vi "WSVCAP SHL FPGA LL Procedure I2C - Receive Byte.vi"(0 "Procedure Step":T1, 1 "Wait Ticks Remaining":u32, 5 "I2C Wait Ticks":u32, 7 "Read Bits Remaining":u8, 9 "Read Bytes Remaining":u8, 11 "error in (no error)":errorcluster, 13 "Socket Mask":u64 format="%012x", 14 "UUT Set (0/1)":u8) -> (3 "Wait Ticks Remaining Out":u32, 4 "Procedure Step Out":T1, 6 "Finished":bool, 8 "Read Bits Remaining Out":u8, 10 "Read Bytes Remaining Out":u8, 15 "error out":errorcluster)   [LabVIEW 2017]
uses:
  Type Defs/WSVCAP SHL Procedure Step Enum.ctl
  Type Defs/WSVCAP SHL FIFO Operation Enum.ctl
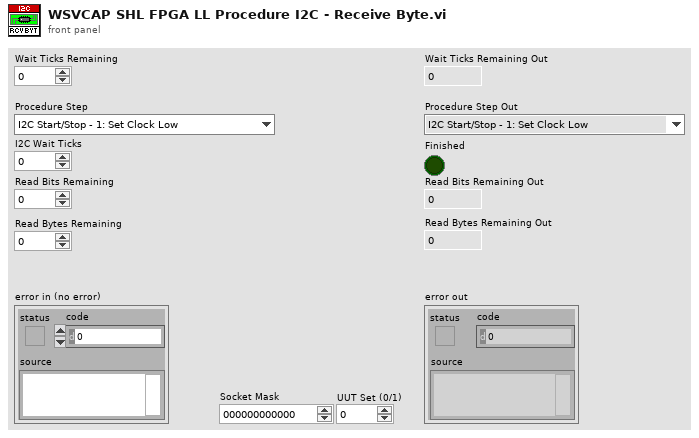
[diagram p1: front panel]
types:
  T1 = typedef "WSVCAP SHL Procedure Step Enum.ctl" = enum16{"I2C Start/Stop - 1: Set Clock Low", "I2C Start/Stop - 2: Wait", "I2C Start/Stop - 3: Set Data I", "I2C Start/Stop - 4: Wait", "I2C Start/Stop - 5: Set Clock High", "I2C Start/Stop - 6: Wait", "I2C Start/Stop - 7: Set Data II", "I2C Start/Stop - 8: Wait", "I2C Start/Stop - 9: Set Clock Low", "I2C Start/Stop - 10: Wait", "I2C Read ACK - 1: Set Clock High", "I2C Read ACK - 2: Wait", "I2C Read ACK - 3: Read ACK Bit", "I2C Read ACK - 4: Wait", "I2C Read ACK - 5: Set Clock Low", "I2C Read ACK - 6: Wait", "I2C Write ACK - 1: Write ACK Bit", "I2C Write ACK - 2: Wait", "I2C Write ACK - 3: Set Clock High", "I2C Write ACK - 4: Wait", "I2C Write ACK - 5: Set Clock Low", "I2C Write ACK - 6: Wait", "I2C Write ACK - 7: Set Data Low", "I2C Send Add - 1: Reset Bits Remaining", "I2C Send Add - 2: Set Data Bit", "I2C Send Add - 3: Wait", "I2C Send Add - 4: Set Clock High", "I2C Send Add - 5: Wait", "I2C Send Add - 6: Set Clock Low", "I2C Send Add - 7: Wait", "I2C Send Add - 8: Check Bits Remaining", "I2C Send Data - 1: Reset Bits Remaining", "I2C Send Data - 2: Load Write Bit from FIFO", "I2C Send Data - 3: Set Data Bit", "I2C Send Data - 4: Wait", "I2C Send Data - 5: Set Clock High", "I2C Send Data - 6: Wait", "I2C Send Data - 7: Set Clock Low", "I2C Send Data - 8: Wait", "I2C Send Data - 9: Check Bits Remaining", "I2C Receive Data - 1: Reset Bits Remaining", "I2C Receive Data - 2: Wait", "I2C Receive Data - 3: Set Clock High", "I2C Receive Data - 4: Wait", "I2C Receive Data - 5: Read Data Bit", "I2C Receive Data - 6: Wait", "I2C Receive Data - 7: Set Clock Low", "I2C Receive Data - 8: Wait", "I2C Receive Data - 9: Check Bits Remaining", "RFFE Send SSC - 1:Set Low", "RFFE Send SSC - 2:Wait", "RFFE Send SSC - 3:Set SDA High", "RFFE Send SSC - 4:Wait", "RFFE Send SSC - 5:Set SDA Low", "RFFE Send SSC - 6:Wait", "RFFE Send Data - 1:Set SCL High", "RFFE Send Data - 2:Wait", "RFFE Send Data - 3:Set SCL Low", "RFFE Send Data - 4:Wait", "RFFE Send Data - 5:Set SCL High (P)", "RFFE Send Data - 6:Wait", "RFFE Send Data - 7:Set SCL Low (P)", "RFFE Send Data - 8:Wait", "RFFE Send Data - 9:Set SCL High (BP)", "RFFE Send Data - 10:Wait", "RFFE Send Data - 11:Set SCL Low (BP)", "RFFE Send Data - 12:Wait", "RFFE Receive Data - 1:Set SCL High", "RFFE Receive Data - 2:Wait", "RFFE Receive Data - 3:Set SCL Low", "RFFE Receive Data - 4:Wait", "RFFE Receive Data - 5:Set SCL High (BP)", "RFFE Receive Data - 6:Wait", "RFFE Receive Data - 7:Set SCL Low (BP)", "RFFE Receive Data - 8:Wait", "RFFE Wait CMD Delay - 1:Wait", "RFFE Clear Lines - 1:Clear", "SRL Write Data - 1:Set SYNC High", "SRL Write Data - 2:Wait SYNC Delay", "SRL Write Data - 3:Set SYNC Low", "SRL Write Data - 4:Set SCLK High", "SRL Write Data - 5:Wait", "SRL Write Data - 6:Set SCLK Low", "SRL Write Data - 7:Wait", "SRL Write Data - 8:Set SYNC High", "SRL Wait CMD Delay - 1:Wait", "SRL Clear Lines - 1:Clear"}
  T2 = typedef "WSVCAP SHL FIFO Operation Enum.ctl" = enum16{"Create FIFO/Memory", "Get Write FIFO Status", "Get Read FIFO Status", "Put Element in Write", "Put Element in Read", "Get Element from Write", "Get Element from Read"}
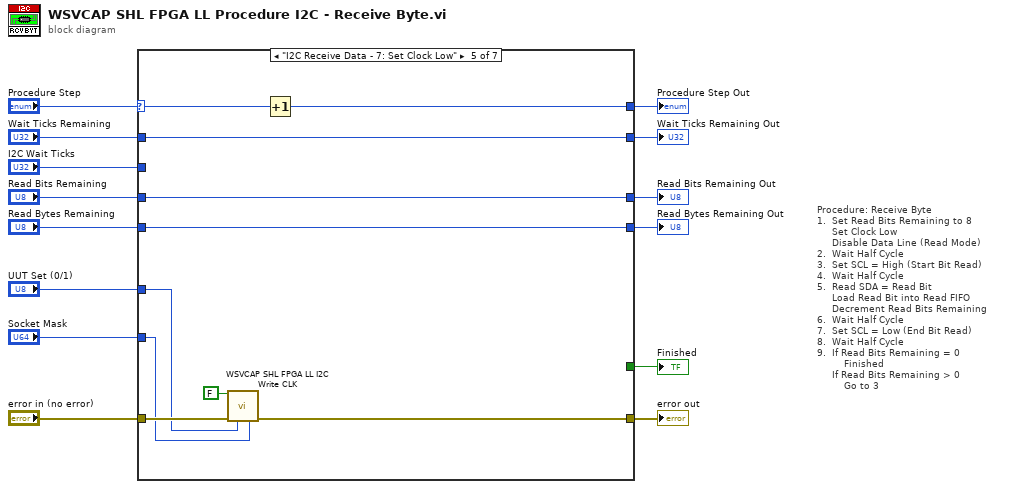
[diagram p0: block diagram]
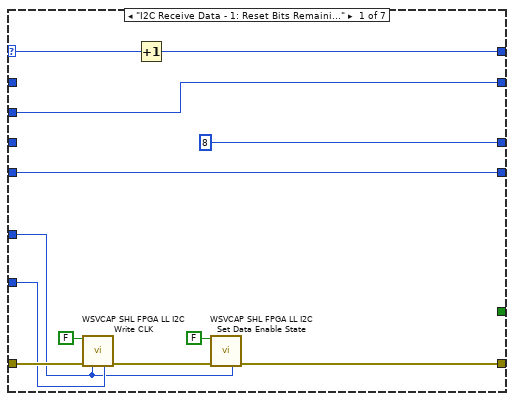
[diagram p2: hidden frame]
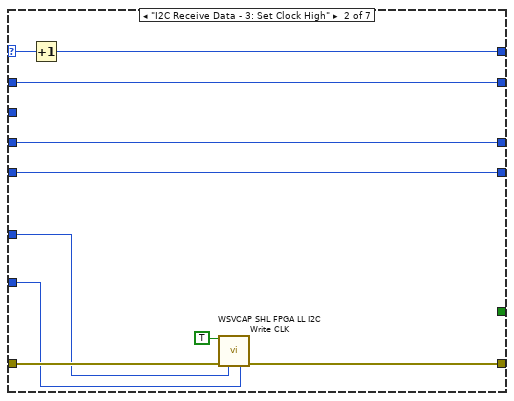
[diagram p3: hidden frame]
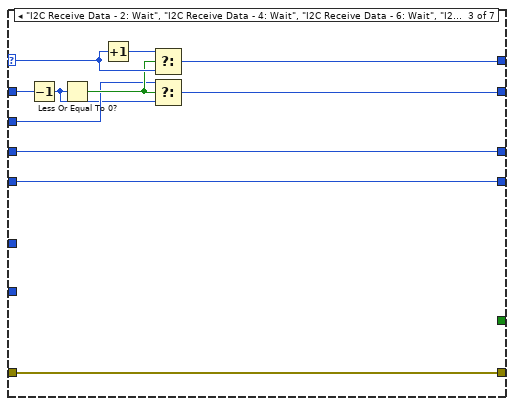
[diagram p4: hidden frame]
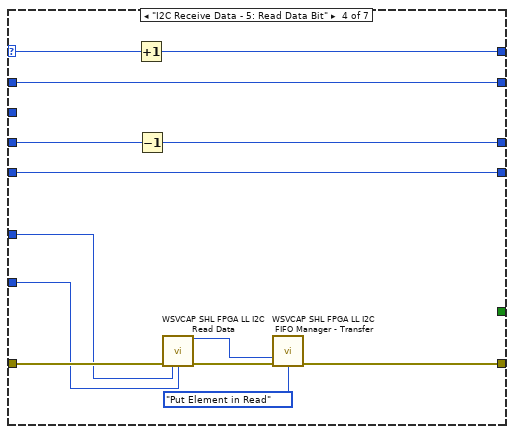
[diagram p5: hidden frame]
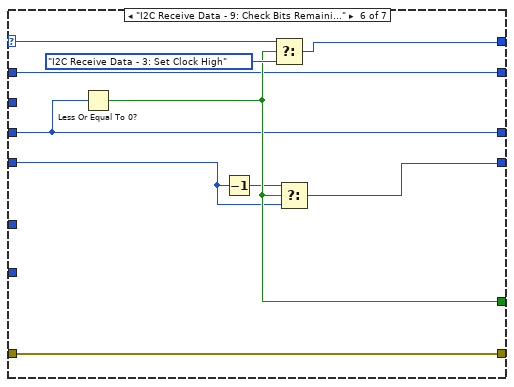
[diagram p6: hidden frame]
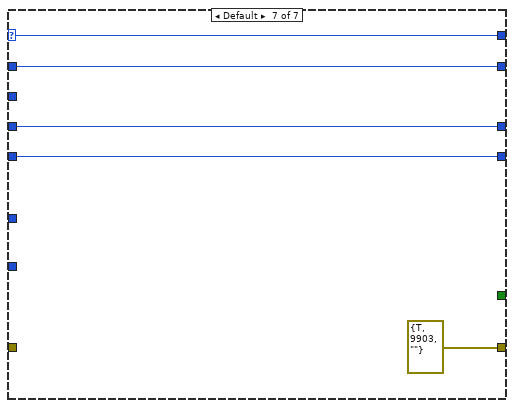
[diagram p7: hidden frame]
diagram:
  # "Procedure: Receive Byte\n1.  Set Read Bits Remaining to 8 \n     Set Clock Low\n     Disable Data Line (Read Mode)\n2.  Wait Half Cycle\n3.  Set SCL = High (Start Bit Read)\n4.  Wait Half Cycle\n5.  Read SDA = Read Bit\n     Load Read Bit into Read FIFO\n     Decrement Read Bits Remaining\n6.  Wait Half Cycle\n7.  Set SCL = Low (End Bit Read)\n8.  Wait Half Cycle\n9.  If Read Bits Remaining = 0\n         Finished\n     If Read Bits Remaining > 0\n         Go to 3"
  n1 = case shown="\"I2C Receive Data - 7: Set Clock Low\"" "Procedure Step" {
    selector: "Procedure Step" -> [w24 w34 w46 w59 w67 w75 w84]
    tunnel: [w22 w35 w44 w57 w69 w80 errorcluster {"status"=TRUE, "code"=9903, "source"=""} ("error IO")] -> w13
    tunnel: "error in (no error)" -> [w26 w36 w44 w60 w70 w80 _]
    tunnel: "Wait Ticks Remaining" -> [_ w30 w47 w50 w64 w72 w83]
    tunnel: "I2C Wait Ticks" -> [w17 _ w42 _ _ _ _]
    tunnel: "Read Bits Remaining" -> [_ w29 w38 w54 w63 w71 w82]
    tunnel: [_ _ _ _ _ w78 _] -> w12
    tunnel: "Socket Mask" -> [w20 w32 _ w53 w66 _ _]
    tunnel: "Read Bytes Remaining" -> [w16 w28 w37 w49 w62 w77 w81]
    tunnel: [w19 w31 w40 w52 w65 w74 w84] -> w11
    tunnel: [w16 w28 w37 w49 w62 w73 w81] -> w10
    tunnel: [w17 w30 w39 w50 w64 w72 w83] -> w3
    tunnel: [u8 8 ("Write Bits Remaining") w29 w38 w51 w63 w71 w82] -> w2
    tunnel: "UUT Set (0/1)" -> [w15 w27 _ w48 w61 _ _]
    frame "I2C Receive Data - 1: Reset Bits Remaining" {
      n2 = call "WSVCAP SHL FPGA LL I2C Write CLK.vi"("Bit In"=FALSE, "error in (no error)"=w26, "UUT Set (0/1 (Legacy)"=w15, "Socket Mask"=w20) -> ("error out"=w23:errorcluster)  [unwired: 11 in]
      n3 = Increment(x=w24) -> (x+1=w19:T1)
      n4 = call "WSVCAP SHL FPGA LL I2C Set Data Enable State.vi"("State"=FALSE, "error in (no error)"=w23, "UUT Set (0/1)"=w15) -> ("error out"=w22:errorcluster)  [unwired: 12 in]
    }
    frame "I2C Receive Data - 3: Set Clock High" {
      n5 = Increment(x=w34) -> (x+1=w31:T1)
      n6 = call "WSVCAP SHL FPGA LL I2C Write CLK.vi"("Bit In"=TRUE, "error in (no error)"=w36, "UUT Set (0/1 (Legacy)"=w27, "Socket Mask"=w32) -> ("error out"=w35:errorcluster)  [unwired: 11 in]
    }
    frame "I2C Receive Data - 2: Wait", "I2C Receive Data - 4: Wait", "I2C Receive Data - 6: Wait", "I2C Receive Data - 8: Wait" {
      n7 = Decrement(x=w47) -> (x-1=w41:u32)
      n8 = Less Or Equal To 0?(x=w41) -> (x <= 0?=w43:bool)
      n9 = Increment(x=w46) -> (x+1=w45:T1)
      n10 = Select(t=w45, s=w43, f=w46) -> (s? t:f=w40:T1)
      n11 = Select(t=w42, s=w43, f=w41) -> (s? t:f=w39:u32)
    }
    frame "I2C Receive Data - 5: Read Data Bit" {
      n12 = Increment(x=w59) -> (x+1=w52:T1)
      n13 = Decrement(x=w54) -> (x-1=w51:u8)
      n14 = call "WSVCAP SHL FPGA LL I2C Read Data.vi"("error in (no error)"=w60, "UUT Set (0-1) (Legacy)"=w48, "Socket Mask"=w53) -> ("Long Word Out (1-Bit for Each Channel)"=w55:u64, "error out"=w58:errorcluster)  [unwired: 11 in]
      n15 = call "WSVCAP SHL FPGA LL I2C FIFO Manager - Transfer.vi"("Long Word In"=w55, "error in (no error)"=w58, "Operation"=WSVCAP_SHL_FIFO_Operation_Enum."Put Element in Read") -> ("error out"=w57:errorcluster)  [unwired: 10 in, 2 out]
    }
    frame "I2C Receive Data - 7: Set Clock Low" {
      n16 = call "WSVCAP SHL FPGA LL I2C Write CLK.vi"("Bit In"=FALSE, "error in (no error)"=w70, "UUT Set (0/1 (Legacy)"=w61, "Socket Mask"=w66) -> ("error out"=w69:errorcluster)  [unwired: 11 in]
      n17 = Increment(x=w67) -> (x+1=w65:T1)
    }
    frame "I2C Receive Data - 9: Check Bits Remaining" {
      n18 = Less Or Equal To 0?(x=w71) -> (x <= 0?=w78:bool)
      n19 = Decrement(x=w77) -> (x-1=w76:u8)
      n20 = Select(t=w75, s=w78, f=WSVCAP_SHL_Procedure_Step_Enum."I2C Receive Data - 3: Set Clock High" ("Procedure Step")) -> (s? t:f=w74:T1)
      n21 = Select(t=w76, s=w78, f=w77) -> (s? t:f=w73:u8)
    }
    frame Default {
    }
  }
  "error out" <- w13
  "Finished" <- w12
  "Procedure Step Out" <- w11
  "Read Bytes Remaining Out" <- w10
  "Wait Ticks Remaining Out" <- w3
  "Read Bits Remaining Out" <- w2
